vi "rSetup.vi"(0 "Socket_000 in":refnum<class "TCPAlerts.lvclass">, 11 "error in (no error)":errorcluster) -> (4 "Socket_000 out":refnum<class "TCPAlerts.lvclass">, 6 "IP Address":string, 8 "Port":u16, 15 "error out":errorcluster)   [LabVIEW 2011, in "TCPAlerts.lvclass"]
uses:
  TCPAlerts.lvclass
  TCPAlerts.lvclass/TCPAlerts.ctl
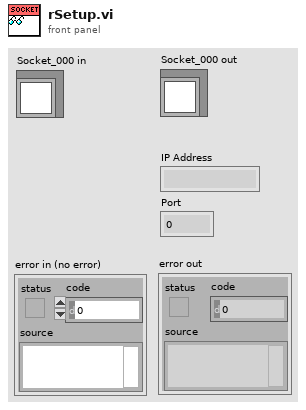
[diagram p1: front panel]
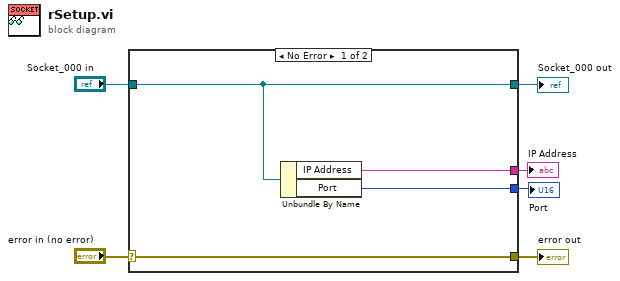
[diagram p0: block diagram]
diagram:
  n1 = case shown="No Error" "error in (no error)" {
    selector: "error in (no error)" -> [w10 w11]
    tunnel: [w10 w11] -> w4
    tunnel: [w9 w12] -> w5
    tunnel: "Socket_000 in" -> [w9 w12]
    tunnel: [w8 _] -> w2
    tunnel: [w7 _] -> w1
    frame No Error {
      n2 = Unbundle By Name(w9) -> ("IP Address"=w8:string, "Port"=w7:u16)
    }
    frame Error {
    }
  }
  "error out" <- w4
  "Socket_000 out" <- w5
  "IP Address" <- w2
  "Port" <- w1
